vi "Comms.vi"(11 "I2CDevRef in":T1 {"Device Address" format="%.0x"}) -> (3 "I2CDevRef out":T1 {"Device Address" format="%.0x"})   [LabVIEW 2013]
uses:
  <vilib>/Rock Robotics/WPI/I2C/WPI_I2CDevRef.ctl
  <vilib>/Rock Robotics/SystemInterfaces/Typedef/FPGA_TypedefDigitalModule.ctl
  Robot Global Data.vi
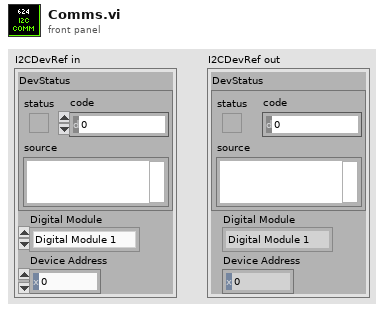
[diagram p1: front panel]
types:
  T1 = typedef "WPI_I2CDevRef.ctl" = cluster{"DevStatus":errorcluster, "Digital Module":T2, "Device Address":u8}
  T2 = typedef "FPGA_TypedefDigitalModule.ctl" = enum16{"Digital Module 1", "Digital Module 2"}
  T3 = enum16{"Shoot Ready", "Shoot", "Hold Ball", "Rollers"}
  T4 = typedef "WPI_DriverStationRobotMode2.ctl" = enum16{"Autonomous Disabled", "Autonomous Enabled", "Teleop Disabled", "Teleop Enabled", "Timeout", "Finish", "Test Disabled", "Test Enabled"}
  T5 = typedef "WPI_DriverStationAllianceInfo.ctl" = enum16{"Red", "Blue", "Invalid"}
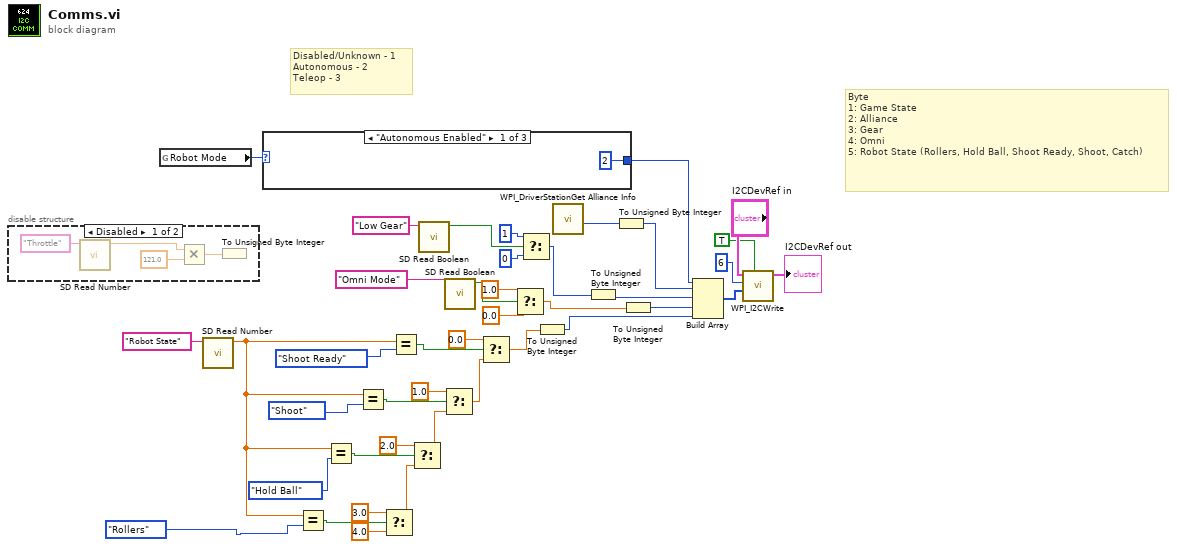
[diagram p0: block diagram]
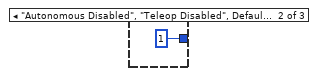
[diagram p3: hidden frame]
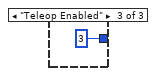
[diagram p4: hidden frame]
diagram:
  # "Byte\n1: Game State\n2: Alliance\n3: Gear\n4: Omni\n5: Robot State (Rollers, Hold Ball, Shoot Ready, Shoot, Catch)"
  # "Disabled/Unknown - 1\nAutonomous - 2\nTeleop - 3"
  n1 = disable-structure shown="Disabled" {
    frame Disabled {
      n2 = call <vilib>:"SD Read Number.vi"("Name"="Throttle") -> ("Numeric"=w42:dbl)  [unwired: 8 in, 2 out]
      n3 = Multiply(x=w42, y=121.0) -> (x*y=w45:dbl)
      n4 = To Unsigned Byte Integer(number=w45) -> ()  [unwired: 1 out]
    }
    frame Enabled {
    }
  }
  n5 = global read "Robot Global Data.vi" "Robot Mode"() -> (w39:T4)
  n6 = call <vilib>:"SD Read Number.vi"("Name"="Robot State") -> ("Numeric"=w19:dbl)  [unwired: 8 in, 2 out]
  n7 = case shown="\"Autonomous Enabled\"" w39 {
    tunnel: [u8 2 u8 1 u8 3] -> w41
    frame "Autonomous Enabled" {
    }
    frame "Autonomous Disabled", "Teleop Disabled", Default {
    }
    frame "Teleop Enabled" {
    }
  }
  n8 = Equal?(x=w19, y=T3."Rollers") -> (x = y?=w27:bool)
  n9 = Equal?(x=w19, y=T3."Hold Ball") -> (x = y?=w29:bool)
  n10 = Equal?(x=w19, y=T3."Shoot") -> (x = y?=w32:bool)
  n11 = Select(t=3.0, s=w27, f=4.0) -> (s? t:f=w26:dbl)
  n12 = Equal?(x=w19, y=T3."Shoot Ready") -> (x = y?=w34:bool)
  n13 = Select(t=2.0, s=w29, f=w26) -> (s? t:f=w28:dbl)
  n14 = call <vilib>:"SD Read Boolean.vi"("Name"="Low Gear") -> ("Boolean"=w10:bool)  [unwired: 8 in, 2 out]
  n15 = Select(t=1.0, s=w32, f=w28) -> (s? t:f=w24:dbl)
  n16 = call <vilib>:"SD Read Boolean.vi"("Name"="Omni Mode") -> ("Boolean"=w11:bool)  [unwired: 8 in, 2 out]
  n17 = Select(t=0.0, s=w34, f=w24) -> (s? t:f=w17:dbl)
  n18 = Select(t=1.0, s=w11, f=0.0) -> (s? t:f=w2:dbl)
  n19 = Select(t=u8 1 ("I2CRegister"), s=w10, f=u8 0) -> (s? t:f=w7:u8)
  n20 = To Unsigned Byte Integer(number=w17) -> (unsigned 8bit integer=w4:u8)
  n21 = call <vilib>:"WPI_DriverStationGet Alliance Info.vi"() -> ("Alliance"=w36:T5)  [unwired: 10 in, 1 out]
  n22 = To Unsigned Byte Integer(number=w7) -> (unsigned 8bit integer=w15:u8)
  n23 = To Unsigned Byte Integer(number=w36) -> (unsigned 8bit integer=w35:u8)
  n24 = To Unsigned Byte Integer(number=w2) -> (unsigned 8bit integer=w3:u8)
  n25 = Build Array(w41, w35, w15, w3, w4) -> (w40:u8[])
  n26 = call <vilib>:"WPI_I2CWrite.vi"("CompatibilityMode"=TRUE, "I2CDataToSend"=w40, "I2CRegister"=u8 6, "I2CDevRef"="I2CDevRef in") -> ("I2CDevRef"=→"I2CDevRef out":T1)  [unwired: 6 in, 1 out]
